vi "runDisplay.vi"(8 "error in (no error)":errorcluster, 11 "DisplayElement.lvclass":refnum<class "DisplayElement.lvclass">) -> (0 "error out":errorcluster, 3 "DisplayElement.lvclass 2":refnum<class "DisplayElement.lvclass">)   [LabVIEW 2020, in "DisplayElement.lvclass"]
uses:
  DisplayElement.lvclass
panel:
  # "Connector Pane"
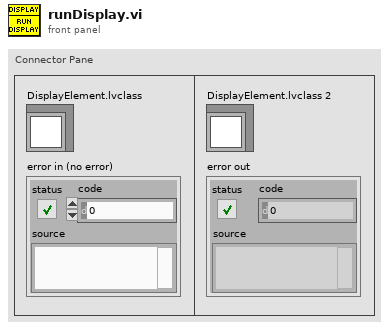
[diagram p1: front panel]
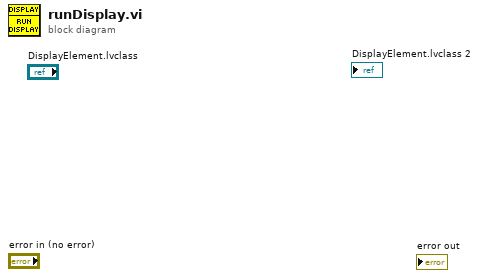
[diagram p0: block diagram]
diagram:
